vi "Variant to Array of Variants.vi"(8 "error in (no error)":errorcluster, 11 "variant":variant) -> (0 "error out":errorcluster, 3 "Array":variant[](array[variant]))   [LabVIEW 2016, in "JSFL Variant Support.lvlib"]
uses:
  JSFL Variant Support.lvlib
  <vilib>/Utility/Data Type/NI_Data Type.lvlib
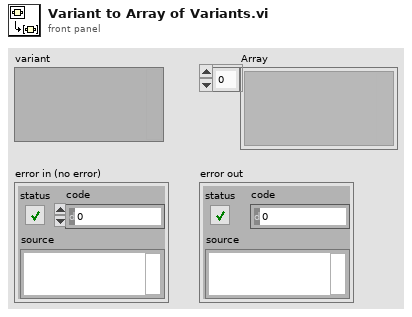
[diagram p1: front panel]
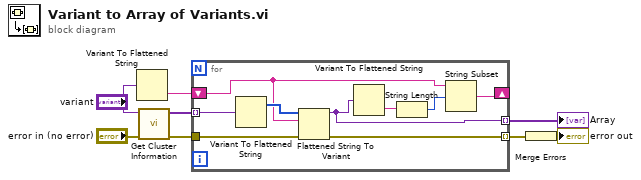
[diagram p0: block diagram]
diagram:
  n1 = Variant To Flattened String(Variant="variant") -> (data string=w1:string)  [unwired: 1 out]
  n2 = call <vilib>:"Get Cluster Information.vi"("error in (no error)"="error in (no error)", "Variant"="variant") -> ("error out"=w3:errorcluster, "Cluster Elements"=w2:variant[])  [unwired: 8 in]
  n3 = for {
    tunnel: w2 -> [w17] mode=indexing
    tunnel: [w15] -> w5 mode=indexing
    shift-right: [w11] -> _
    shift-left: w1 -> [w14]
    tunnel: w3 -> [w10]
    tunnel: [w9] -> w4 mode=indexing
    n4 = Variant To Flattened String(Variant=w17) -> (1:w16:i16[])  [unwired: 1 out]
    n5 = Flattened String To Variant(4:w10, 6:w14, 7:w16) -> (0:w9:errorcluster, 3:w15:variant)
    n6 = Variant To Flattened String(Variant=w15) -> (data string=w13:string)  [unwired: 1 out]
    n7 = String Length(string=w13) -> (length=w12:i32)
    n8 = String Subset(string=w14, offset (0)=w12) -> (substring=w11:string)  [unwired: 1 in]
  }
  "Array" <- w5
  n9 = Merge Errors(w4) -> (→"error out":errorcluster)
